vi "Hardware Device Get Info.vi"(8 "error in (no error)":errorcluster, 11 "AI in":refnum<class "AI.lvclass">) -> (0 "error out":errorcluster, 3 "AI out":refnum<class "AI.lvclass">)   [LabVIEW 2023, in "HardwareAbstractionLayer_LVOOP.lvlib" / "AI.lvclass"]
uses:
  AI.lvclass
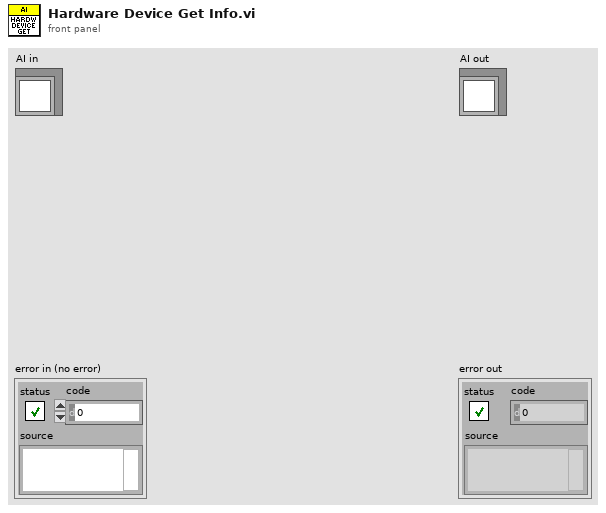
[diagram p1: front panel]
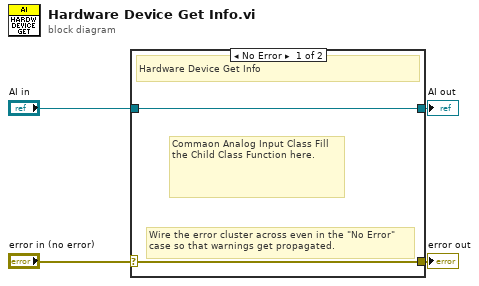
[diagram p0: block diagram]
diagram:
  n1 = case shown="No Error" "error in (no error)" {
    selector: "error in (no error)" -> [w5 w8]
    tunnel: [w5 w8] -> w3
    tunnel: [w6 w7] -> w1
    tunnel: "AI in" -> [w6 w7]
    frame No Error {
      # "Commaon Analog Input Class Fill the Child Class Function here."
      # "Wire the error cluster across even in the \"No Error\"\ncase so that warnings get propagated."
      # "Hardware Device Get Info"
    }
    frame Error {
    }
  }
  "error out" <- w3
  "AI out" <- w1
